vi "GetProperties.vi"(8 "error in":errorcluster, 11 "Knob in":refnum<class "Knob.lvclass">) -> (0 "error out":errorcluster, 3 "Knob out":refnum<class "Knob.lvclass">)   [LabVIEW 2014, in "Knob.lvclass"]
uses:
  Knob.lvclass
  Knob.lvclass/Knob.ctl
  NumericWithScale/NumericWithScale.lvclass
  RotaryColorScale/RotaryColorScale.lvclass
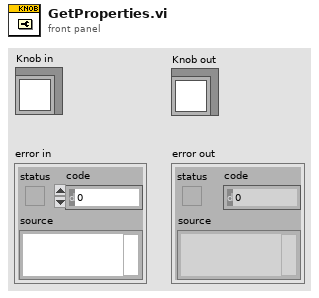
[diagram p1: front panel]
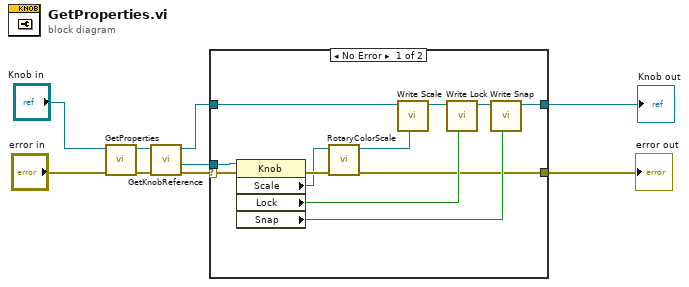
[diagram p0: block diagram]
diagram:
  n1 = call-parent "GetProperties.vi"("error in"="error in", "NumericWithScale in"="Knob in") -> ("error out"=w6:errorcluster, "NumericWithScale out"=w7:refnum<class "Knob.lvclass">)  [unwired: 8 in]
  n2 = call "GetKnobReference.vi"("error in"=w6, "Knob in"=w7) -> ("error out"=w5:errorcluster, "knob reference"=w4:refnum<vi>, "Knob out"=w3:refnum<class "Knob.lvclass">)  [unwired: 7 in]
  n3 = case shown="No Error" w5 {
    selector: w5 -> [w20 w22]
    tunnel: w4 -> [w21 _]
    tunnel: [w12 w23] -> w1
    tunnel: w3 -> [w11 w23]
    tunnel: [w10 w22] -> w2
    frame No Error {
      n4 = property class="Knob"(reference=w21, error in=w20) -> (error out=w19:errorcluster, "Scale"=w18:refnum<vi>, "Lock"=w15:bool, "Snap"=w13:bool)  [unwired: 1 out]
      n5 = call "RotaryColorScale.vi"("error in"=w19, "Gen Refnum"=w18) -> ("error out"=w10:errorcluster, "RotaryColorScale out"=w17:refnum<class "RotaryColorScale.lvclass">)  [unwired: 8 in]
      n6 = call "Write Scale.vi"("Scale"=w17, "Knob in"=w11) -> ("Knob out"=w16:refnum<class "Knob.lvclass">)  [unwired: 7 in]
      n7 = call "Write Lock.vi"("Lock"=w15, "Knob in"=w16) -> ("Knob out"=w14:refnum<class "Knob.lvclass">)  [unwired: 7 in]
      n8 = call "Write Snap.vi"("Snap"=w13, "Knob in"=w14) -> ("Knob out"=w12:refnum<class "Knob.lvclass">)  [unwired: 7 in]
    }
    frame Error {
    }
  }
  "error out" <- w2
  "Knob out" <- w1
